vi "tensile_strength - Copy_debug.vi"(8 "Sampling rate":dbl=1000.0, 9 "error in (no error)":errorcluster, 10 "Sensor":tag="SimDev1/ai0:1", 11 "VISA Refnum in":refnum<visa-resource-name>) -> (1 "error out":errorcluster, 3 "VISA Refnum out":refnum<visa-resource-name>)   [LabVIEW 2020]
uses:
  <vilib>/DAQmx/read.llb/DAQmx Read (Analog 1D DBL NChan 1Samp).vi
  <vilib>/DAQmx/create/channels.llb/DAQmx Create Channel (AI-Voltage-Basic).vi
  <vilib>/DAQmx/configure/timing.llb/DAQmx Timing (Sample Clock).vi
  <vilib>/DAQmx/miscellaneous.llb/DAQmx Fill In Error Info.vi
panel:
  out "t = 3 - 0":dbl
  out "t = 1 - 0":dbl
  out "String":string
  in  "Lower limit for positioning":dbl
  out "distance value \n(changing)":dbl
  out "initial value(fixed)":dbl
  out "State indicator":u32
  in  "Upper limit for force":dbl
  in  "Upper limit for position":dbl
  in  "Emergency stop program(Long press)":bool
  out "Read":string
  in  "Stop motor":bool
  in  "Filename without ending":string="test"
  in  "File path":path=path "d:/temp"
  in  "Speed Write in mircometer/sec":string
  in  "Start Program":bool
  out "Numeric 3":i32
  in  "End the program":bool
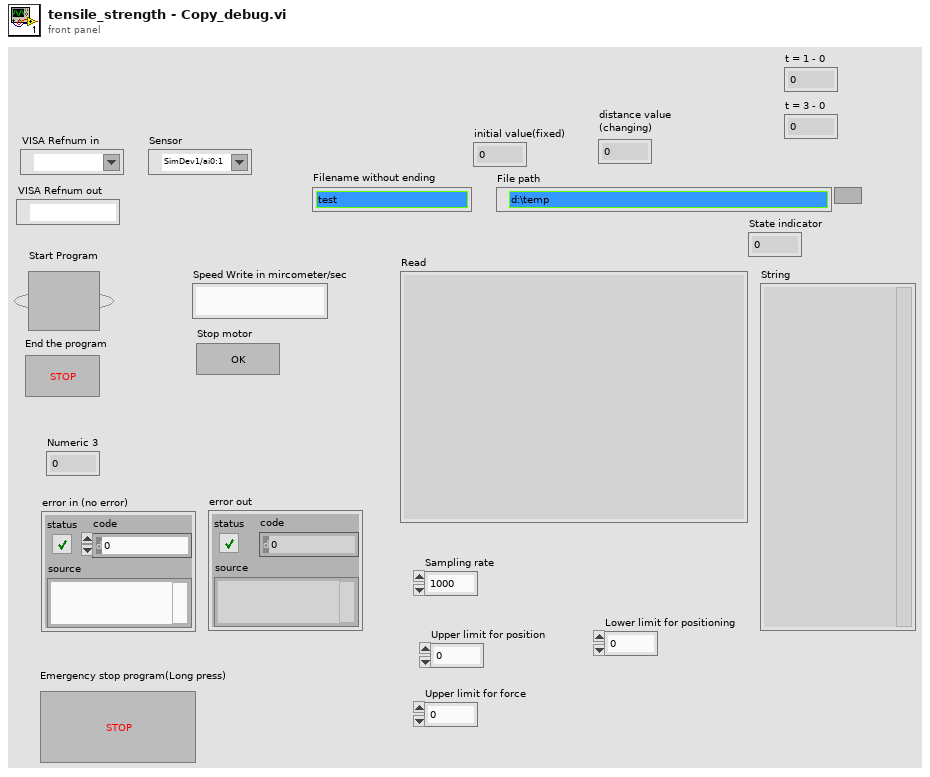
[diagram p1: front panel]
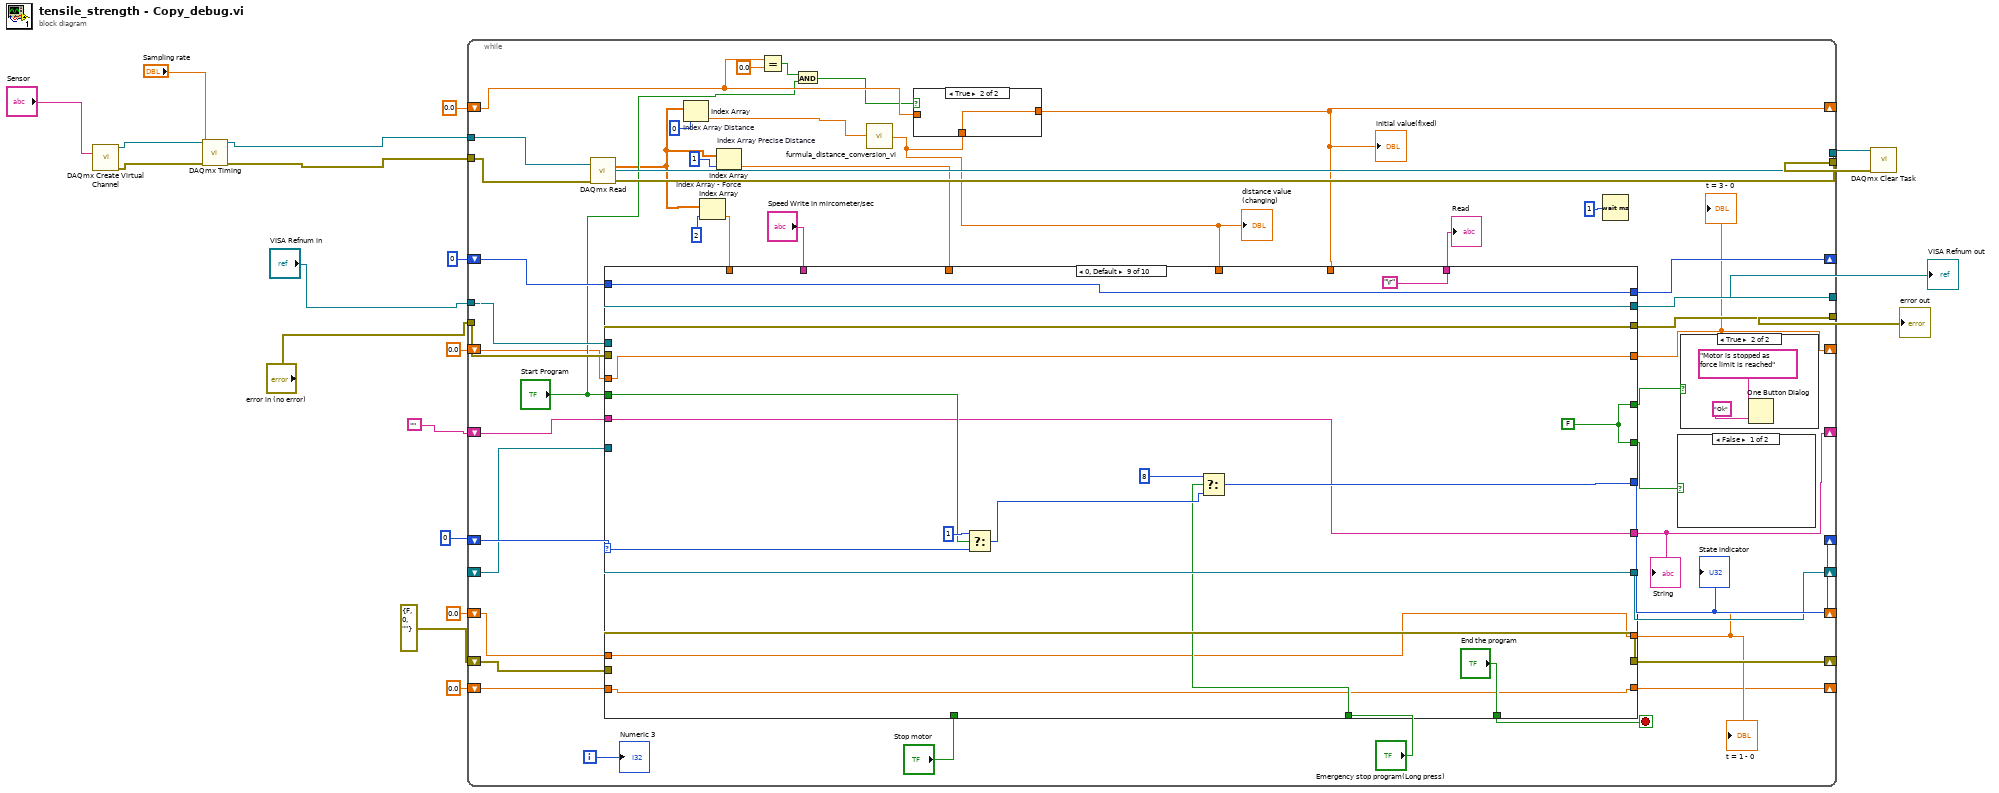
[diagram p0: block diagram]
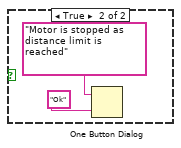
[diagram p2: hidden frame]
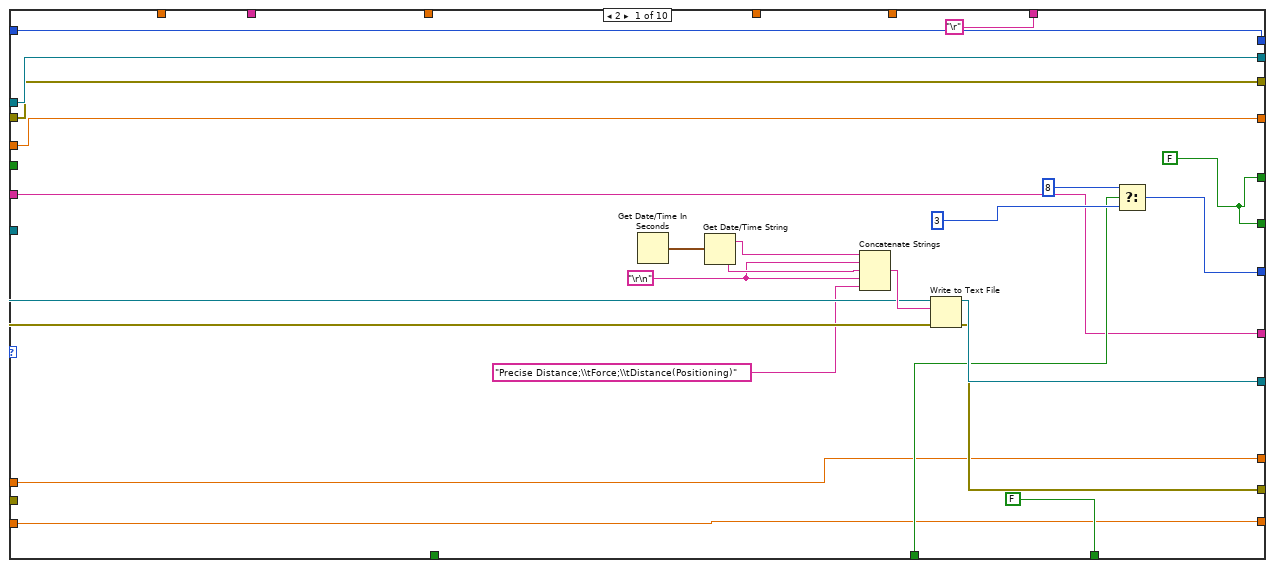
[diagram p5: hidden frame]
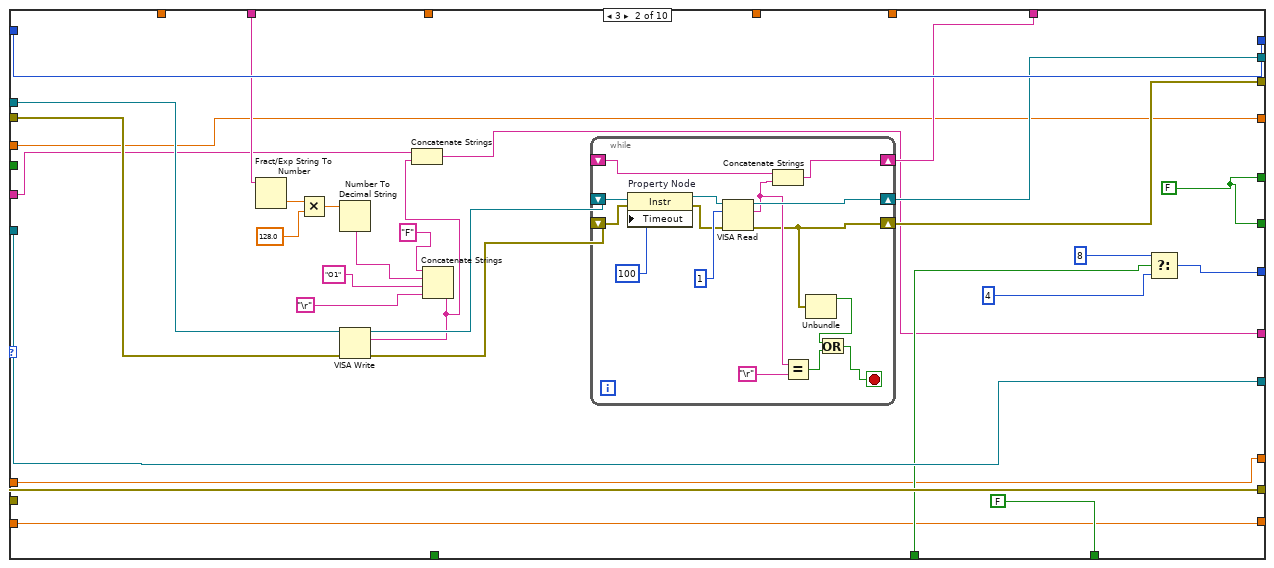
[diagram p6: hidden frame]
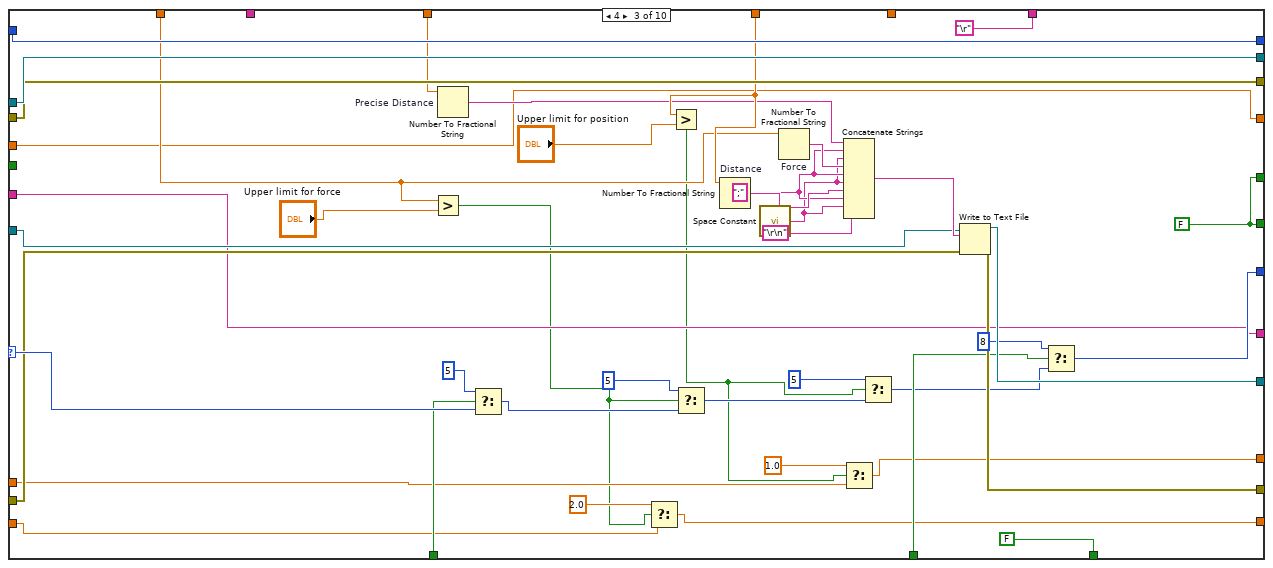
[diagram p7: hidden frame]
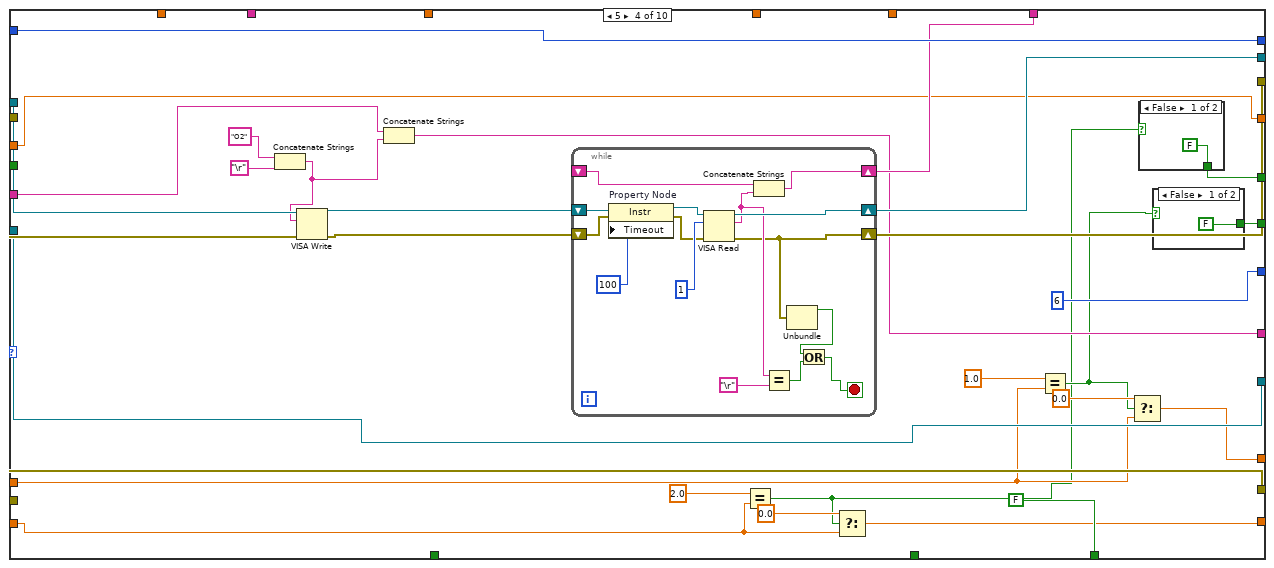
[diagram p8: hidden frame]
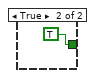
[diagram p9: hidden frame]
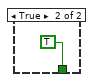
[diagram p10: hidden frame]
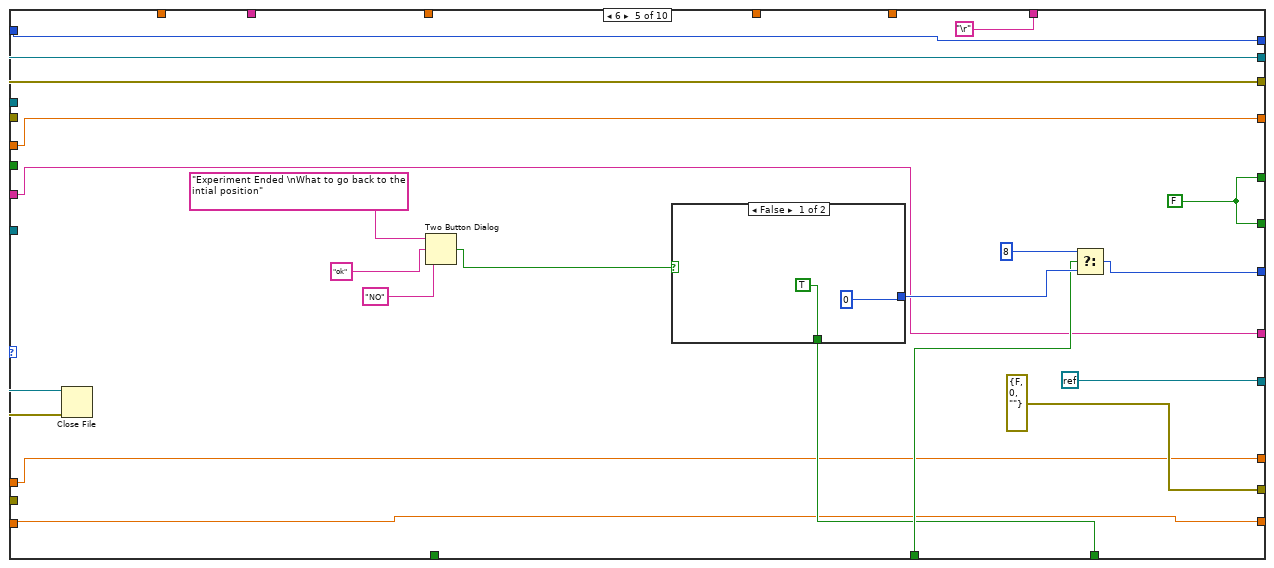
[diagram p11: hidden frame]
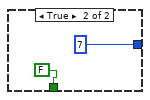
[diagram p12: hidden frame]
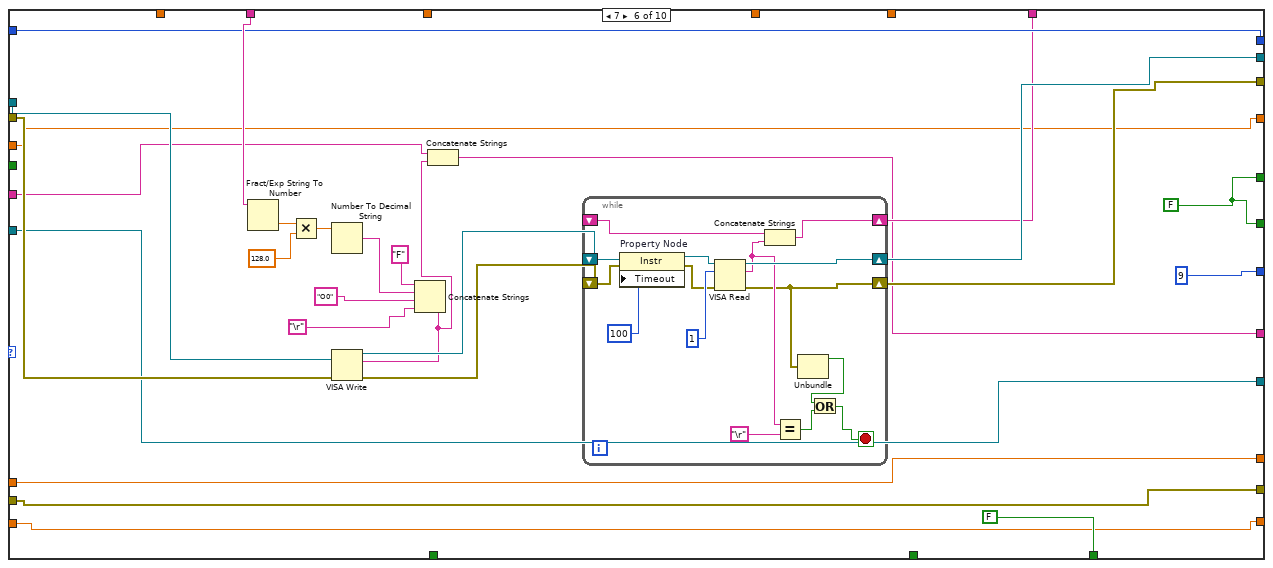
[diagram p13: hidden frame]
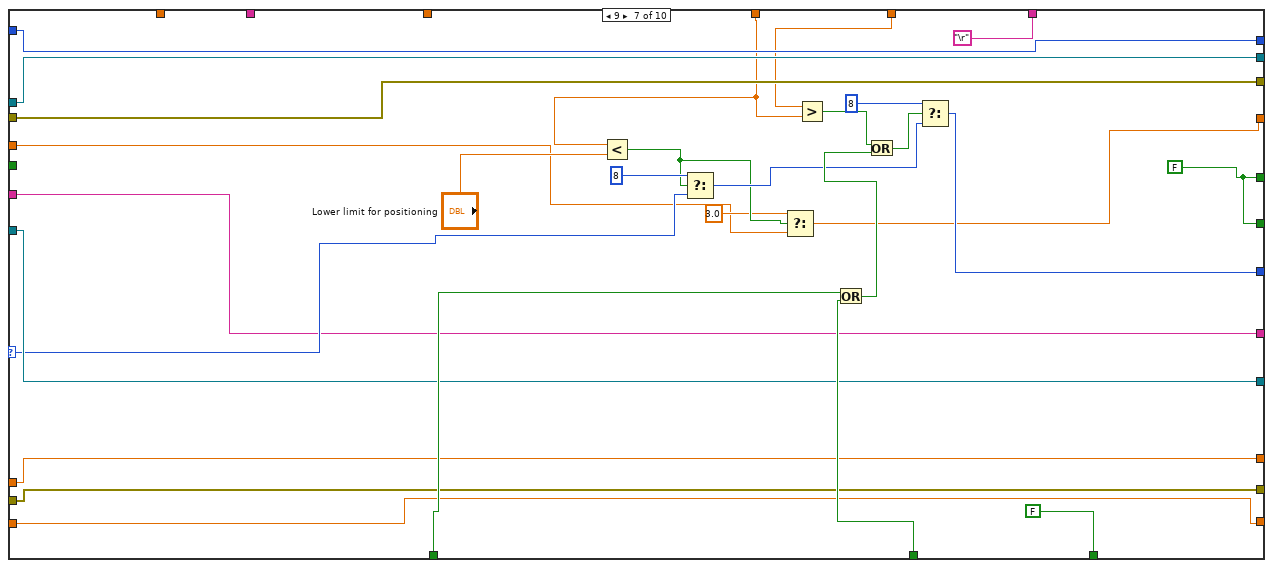
[diagram p14: hidden frame]
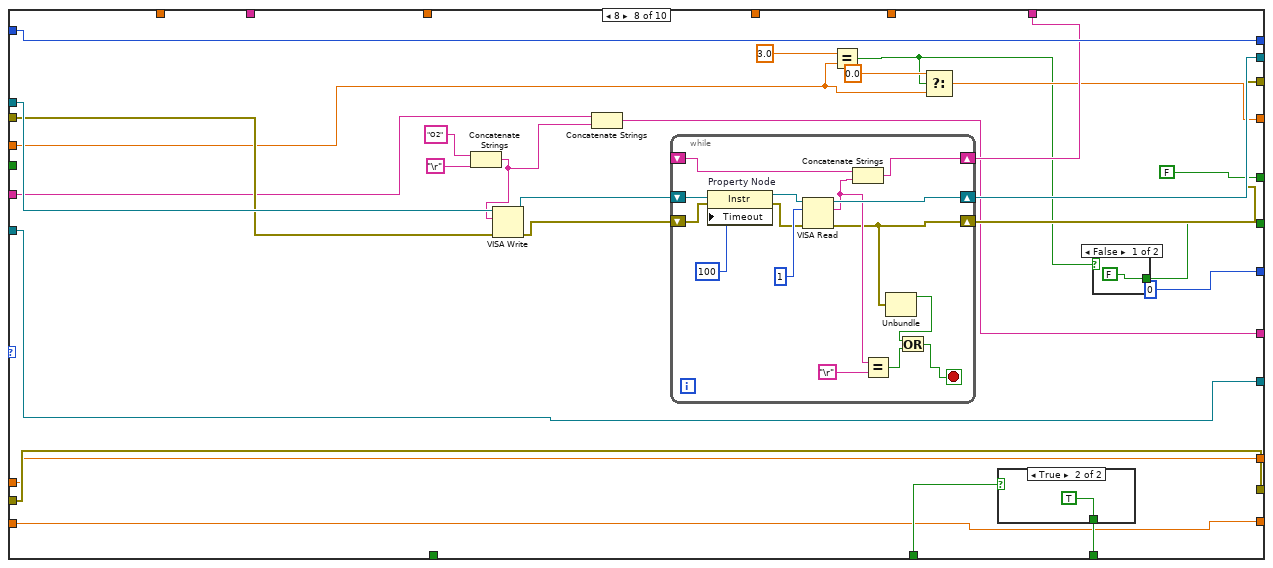
[diagram p15: hidden frame]
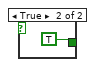
[diagram p16: hidden frame]
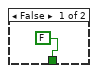
[diagram p17: hidden frame]
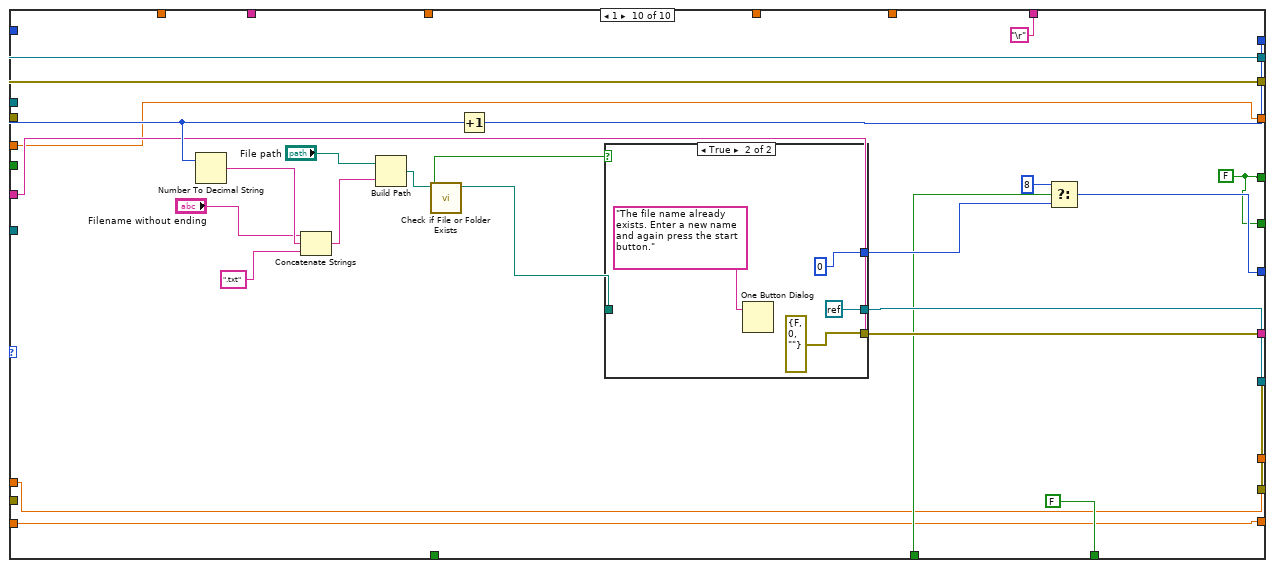
[diagram p18: hidden frame]
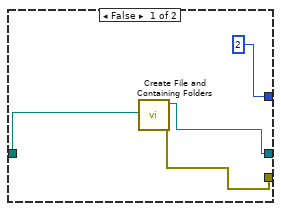
[diagram p19: hidden frame]
diagram:
  n1 = call-poly <vilib>:"DAQmx Create Virtual Channel.vi"("physical channels"="Sensor") -> ("task out"=w17:refnum<k21>, "error out"=w16:errorcluster)  [unwired: 13 in]
  n2 = call-poly <vilib>:"DAQmx Timing.vi"("task/channels in"=w17, "rate"="Sampling rate", "error in"=w16) -> ("task out"=w6:refnum<k21>, "error out"=w5:errorcluster)  [unwired: 11 in]
  n3 = while {
    tunnel: "VISA Refnum in" -> [w67]
    tunnel: "error in (no error)" -> [w66]
    tunnel: [w65] -> w8
    tunnel: [w64] -> w9
    shift-right: [w61] -> _
    shift-left: 0 -> [w63]
    shift-right: [w60] -> _
    shift-left: errorcluster {"status"=FALSE, "code"=0, "source"=""} ("error out") -> [w59]
    shift-right: [w58] -> _
    shift-left: 0 -> [w57]
    shift-right: [w56] -> _
    shift-left: _ -> [w55]
    tunnel: w6 -> [w53]
    tunnel: w5 -> [w54]
    tunnel: [w52] -> w15
    tunnel: [w51] -> w14
    shift-right: [w32] -> _
    shift-left: 0.0 -> [w46]
    shift-right: [w29] -> _
    shift-left: "" -> [w30]
    shift-right: [w28] -> _
    shift-left: 0.0 -> [w27]
    shift-right: [w26] -> _
    shift-left: 0.0 ("t") -> [w25]
    shift-right: [w24] -> _
    shift-left: 0.0 ("t") -> [w23]
    i -> [w62]
    stop <- w34 stop-if-true
    n4 = call-poly <vilib>:"DAQmx Read.vi"("task/channels in"=w53, "error in"=w54) -> ("task out"=w51:refnum<k21>, "data"=w37:dbl[], "error out"=w52:errorcluster)  [unwired: 11 in]
    n5 = Index Array "Index Array Distance"(array=w37, index=0) -> (element=w21:dbl)
    n6 = Index Array "Index Array - Force"(array=w37, index=2) -> (element=w47:dbl)
    n7 = Index Array "Index Array Precise Distance"(array=w37, index=1) -> (element=w35:dbl)
    n8 = Equal?(x=w46, y=0.0) -> (x = y?=w44:bool)
    n9 = And(x=w44, y="Start Program") -> (x .and. y?=w42:bool)
    n10 = call "furmula_distance_conversion_vi.vi"("Schieberegler"=w21) -> ("Numeric"=w22:dbl)
    "distance value \n(changing)" <- w22
    n11 = case shown="True" w42 {
      tunnel: w46 -> [w72 _]
      tunnel: w22 -> [_ w73]
      tunnel: [w72 w73] -> w32
      frame False {
      }
      frame True {
      }
    }
    "initial value(fixed)" <- w32
    n12 = case shown="0, Default" w63 {
      selector: w63 -> [_ _ w185 _ _ _ w313 _ w393 _]
      tunnel: w67 -> [w85 w127 w174 w214 w252 w282 w321 w353 w395 w408]
      tunnel: w66 -> [w84 w126 w173 w213 w251 w281 w320 w352 w394 w407]
      tunnel: [w84 w113 w173 w207 w251 w276 w320 w346 w394 w407] -> w65
      tunnel: [w85 w112 w174 w208 w252 w277 w321 w347 w395 w408] -> w64
      tunnel: [w81 w107 w154 u32 6 ("byte count") w242 9 w324 0 w384 w402] -> w61
      tunnel: [w89 w125 w178 w215 errorcluster {"status"=FALSE, "code"=0, "source"=""} ("error out") w278 w317 w349 w391 w409] -> w60
      tunnel: w59 -> [w91 w125 w177 w215 w256 w278 w317 w349 w391 _]
      tunnel: [FALSE FALSE FALSE FALSE w239 FALSE FALSE w344 "End the program" FALSE] -> w34
      tunnel: [w86 w122 w175 w206 w250 w275 w322 w351 w388 w412] -> w58
      tunnel: w57 -> [w86 w122 w175 w206 w250 w275 w322 w351 w388 w413]
      tunnel: [w90 w123 w179 w204 refnum<k0> refnum w279 w318 w350 w389 w410] -> w56
      tunnel: w55 -> [w92 w123 w172 w204 w255 w279 w318 w350 w389 _]
      tunnel: "Speed Write in mircometer/sec" -> [_ w118 _ _ _ w280 _ _ _ _]
      tunnel: w47 -> [_ _ w164 _ _ _ _ _ _ _]
      tunnel: w22 -> [_ _ w166 _ _ _ w303 _ _ _]
      tunnel: "Start Program" -> [_ _ _ _ _ _ _ _ w387 _]
      tunnel: w32 -> [_ _ _ _ _ _ w304 _ _ _]
      tunnel: ["\r" w111 "\r" w203 "\r" w273 "\r" w348 "\r" "\r"] -> w41
      tunnel: [w78 w106 w144 w197 w240 w267 w308 FALSE w381 w401] -> w40
      tunnel: "Stop motor" -> [_ _ w158 _ _ _ w326 _ _ _]
      tunnel: "Emergency stop program(Long press)" -> [w79 w109 w156 _ w241 _ w327 w343 w382 w404]
      tunnel: w35 -> [_ _ w165 _ _ _ _ _ _ _]
      tunnel: [w78 w106 w144 w193 w240 w267 w308 w332 w381 w401] -> w33
      tunnel: w30 -> [w77 w102 w153 w201 w238 w266 w312 w339 w380 w400]
      tunnel: [w77 w101 w153 w199 w238 w264 w312 w340 w380 w400] -> w29
      tunnel: [w76 w100 w152 w194 w237 w263 w311 w338 w379 w399] -> w28
      tunnel: w27 -> [w76 w100 w151 w195 w237 w263 w311 w338 w379 w399]
      tunnel: [w75 w99 w147 w189 w236 w262 w310 w337 w378 w398] -> w26
      tunnel: w25 -> [w75 w99 w146 w190 w236 w262 w310 w337 w378 w398]
      tunnel: [w74 w98 w143 w186 w235 w261 w306 w334 w377 w397] -> w24
      tunnel: w23 -> [w74 w98 w143 w186 w235 w261 w305 w331 w377 w397]
      frame 2 {
        w78 = FALSE
        w94 = "\r\n"
        n13 = Get Date/Time In Seconds() -> (seconds since 1Jan1904=w97:timestamp)
        n14 = Get Date/Time String(seconds (now)=w97) -> (date string=w96:string, time string=w95:string)  [unwired: 2 in]
        n15 = Concatenate Strings(w96, w94, w95, w94, "Precise Distance;\\tForce;\\tDistance(Positioning)" ("string")) -> (w93:string)
        n16 = Write to Text File(file (use dialog)=w92, text=w93, error in=w91) -> (refnum out=w90:refnum<file>, error out=w89:errorcluster)  [unwired: 1 in, 1 out]
        n17 = Select(t=8, s=w79, f=3) -> (s? t:f=w81:i32)
      }
      frame 3 {
        w106 = FALSE
        n18 = Fract/Exp String To Number(string=w118) -> (number=w120:dbl)  [unwired: 3 in, 1 out]
        n19 = Multiply(x=w120, y=128.0) -> (x*y=w121:dbl)
        n20 = Number To Decimal String(number=w121) -> (decimal integer string=w105:string)  [unwired: 1 in]
        n21 = Concatenate Strings("F" ("string"), w105, "O1" ("string"), "\r") -> (w103:string)
        n22 = VISA Write(VISA resource name=w127, write buffer=w103, error in (no error)=w126) -> (VISA resource name out=w114:refnum<visa-resource-name>, error out=w115:errorcluster)  [unwired: 1 out]
        n23 = Concatenate Strings(w102, w103) -> (w101:string)
        n24 = while {
          shift-right: [w129] -> w113
          shift-left: w115 -> [w132]
          shift-right: [w142] -> w112
          shift-left: w114 -> [w134]
          shift-right: [w139] -> w111
          shift-left: _ -> [w140]
          stop <- w135 stop-if-true
          n25 = property on="Property Node" class="Instr"(reference=w134, error in=w132, "Timeout"=u32 100 ("General Settings:Timeout Value")) -> (reference out=w133:refnum<visa-resource-name>, error out=w131:errorcluster)
          n26 = VISA Read(VISA resource name=w133, byte count=u32 1, error in (no error)=w131) -> (VISA resource name out=w142:refnum<visa-resource-name>, read buffer=w138:string, error out=w129:errorcluster)  [unwired: 1 out]
          n27 = Concatenate Strings(w140, w138) -> (w139:string)
          n28 = Equal?(x=w138, y="\r") -> (x = y?=w136:bool)
          n29 = Unbundle(w129) -> ("status"=w128:bool)  [unwired: 2 out]
          n30 = Or(x=w128, y=w136) -> (x .or. y?=w135:bool)
        }
        n31 = Select(t=8, s=w109, f=u32 4 ("byte count")) -> (s? t:f=w107:u32)
      }
      frame 4 {
        w144 = FALSE
        w162 = ";"
        n32 = Greater?(x=w164, y="Upper limit for force") -> (0:w145:bool)
        n33 = Number To Fractional String "Precise Distance"(number=w165) -> (F-format string=w163:string)  [unwired: 3 in]
        n34 = Select(t=u32 5, s=w158, f=w185) -> (s? t:f=w171:u32)
        n35 = Select(t=2.0, s=w145, f=w146) -> (s? t:f=w147:dbl)
        n36 = Greater?(x=w166, y="Upper limit for position") -> (0:w149:bool)
        n37 = Select(t=u32 5, s=w145, f=w171) -> (s? t:f=w170:u32)
        n38 = Number To Fractional String "Distance"(number=w166) -> (F-format string=w182:string)  [unwired: 3 in]
        n39 = call <vilib>:"Space Constant.vi"() -> ("String"=w161:string)
        n40 = Number To Fractional String "Force"(number=w164) -> (F-format string=w183:string)  [unwired: 3 in]
        n41 = Concatenate Strings(w163, w162, w161, w183, w162, w161, w182, w162, w161, "\r\n") -> (w180:string)
        n42 = Select(t=1.0, s=w149, f=w151) -> (s? t:f=w152:dbl)
        n43 = Select(t=u32 5, s=w149, f=w170) -> (s? t:f=w155:u32)
        n44 = Write to Text File(file (use dialog)=w172, text=w180, error in=w177) -> (refnum out=w179:refnum<file>, error out=w178:errorcluster)  [unwired: 1 in, 1 out]
        n45 = Select(t=8, s=w156, f=w155) -> (s? t:f=w154:u32)
      }
      frame 5 {
        n46 = Concatenate Strings("O2" ("write buffer"), "\r") -> (w200:string)
        n47 = VISA Write(VISA resource name=w214, write buffer=w200, error in (no error)=w213) -> (VISA resource name out=w211:refnum<visa-resource-name>, error out=w212:errorcluster)  [unwired: 1 out]
        n48 = Concatenate Strings(w201, w200) -> (w199:string)
        n49 = while {
          shift-right: [w221] -> w207
          shift-left: w212 -> [w224]
          shift-right: [w234] -> w208
          shift-left: w211 -> [w226]
          shift-right: [w231] -> w203
          shift-left: _ -> [w232]
          stop <- w227 stop-if-true
          n50 = property on="Property Node" class="Instr"(reference=w226, error in=w224, "Timeout"=u32 100 ("General Settings:Timeout Value")) -> (reference out=w225:refnum<visa-resource-name>, error out=w223:errorcluster)
          n51 = VISA Read(VISA resource name=w225, byte count=u32 1, error in (no error)=w223) -> (VISA resource name out=w234:refnum<visa-resource-name>, read buffer=w230:string, error out=w221:errorcluster)  [unwired: 1 out]
          n52 = Concatenate Strings(w232, w230) -> (w231:string)
          n53 = Equal?(x=w230, y="\r") -> (x = y?=w228:bool)
          n54 = Unbundle(w221) -> ("status"=w220:bool)  [unwired: 2 out]
          n55 = Or(x=w220, y=w228) -> (x .or. y?=w227:bool)
        }
        n56 = Equal?(x=2.0, y=w190) -> (x = y?=w187:bool)
        n57 = Select(t=0.0, s=w187, f=w190) -> (s? t:f=w189:dbl)
        n58 = Equal?(x=1.0, y=w195) -> (x = y?=w188:bool)
        n59 = Select(t=0.0, s=w188, f=w195) -> (s? t:f=w194:dbl)
        n60 = case shown="False" w187 {
          tunnel: [FALSE TRUE] -> w197
          frame False {
          }
          frame True {
          }
        }
        n61 = case shown="False" w188 {
          tunnel: [FALSE TRUE] -> w193
          frame False {
          }
          frame True {
          }
        }
      }
      frame 6 {
        w240 = FALSE
        n62 = Close File(refnum=w255, error in=w256) -> ()  [unwired: 2 out]
        n63 = Two Button Dialog(message="Experiment Ended \nWhat to go back to the intial position", 1:"NO" ("F button name (\"Cancel\")"), 2:"ok" ("T button name (\"OK\")")) -> (T button?=w245:bool)
        n64 = case shown="False" w245 {
          tunnel: [u32 0 ("byte count") u32 7 ("byte count")] -> w243
          tunnel: [TRUE FALSE] -> w239
          frame False {
          }
          frame True {
          }
        }
        n65 = Select(t=8, s=w241, f=w243) -> (s? t:f=w242:u32)
      }
      frame 7 {
        w267 = FALSE
        n66 = Fract/Exp String To Number(string=w280) -> (number=w286:dbl)  [unwired: 3 in, 1 out]
        n67 = Multiply(x=w286, y=128.0) -> (x*y=w287:dbl)
        n68 = Number To Decimal String(number=w287) -> (decimal integer string=w268:string)  [unwired: 1 in]
        n69 = Concatenate Strings("F" ("string"), w268, "O0" ("string"), "\r") -> (w265:string)
        n70 = VISA Write(VISA resource name=w282, write buffer=w265, error in (no error)=w281) -> (VISA resource name out=w283:refnum<visa-resource-name>, error out=w284:errorcluster)  [unwired: 1 out]
        n71 = Concatenate Strings(w266, w265) -> (w264:string)
        n72 = while {
          shift-right: [w289] -> w276
          shift-left: w284 -> [w292]
          shift-right: [w302] -> w277
          shift-left: w283 -> [w294]
          shift-right: [w299] -> w273
          shift-left: _ -> [w300]
          stop <- w295 stop-if-true
          n73 = property on="Property Node" class="Instr"(reference=w294, error in=w292, "Timeout"=u32 100 ("General Settings:Timeout Value")) -> (reference out=w293:refnum<visa-resource-name>, error out=w291:errorcluster)
          n74 = VISA Read(VISA resource name=w293, byte count=u32 1, error in (no error)=w291) -> (VISA resource name out=w302:refnum<visa-resource-name>, read buffer=w298:string, error out=w289:errorcluster)  [unwired: 1 out]
          n75 = Concatenate Strings(w300, w298) -> (w299:string)
          n76 = Equal?(x=w298, y="\r") -> (x = y?=w296:bool)
          n77 = Unbundle(w289) -> ("status"=w288:bool)  [unwired: 2 out]
          n78 = Or(x=w288, y=w296) -> (x .or. y?=w295:bool)
        }
      }
      frame 9 {
        w308 = FALSE
        n79 = Less?(x=w303, y="Lower limit for positioning") -> (x < y?=w309:bool)
        n80 = Select(t=u32 8, s=w309, f=w313) -> (s? t:f=w315:u32)
        n81 = Select(t=3.0, s=w309, f=w305) -> (s? t:f=w306:dbl)
        n82 = Greater?(x=w304, y=w303) -> (0:w329:bool)
        n83 = Or(x=w326, y=w327) -> (x .or. y?=w325:bool)
        n84 = Or(x=w329, y=w325) -> (x .or. y?=w328:bool)
        n85 = Select(t=u32 8, s=w328, f=w315) -> (s? t:f=w324:u32)
      }
      frame 8 {
        n86 = Concatenate Strings("O2" ("write buffer"), "\r") -> (w341:string)
        n87 = VISA Write(VISA resource name=w353, write buffer=w341, error in (no error)=w352) -> (VISA resource name out=w356:refnum<visa-resource-name>, error out=w357:errorcluster)  [unwired: 1 out]
        n88 = Concatenate Strings(w339, w341) -> (w340:string)
        n89 = while {
          shift-right: [w363] -> w346
          shift-left: w357 -> [w366]
          shift-right: [w376] -> w347
          shift-left: w356 -> [w368]
          shift-right: [w373] -> w348
          shift-left: _ -> [w374]
          stop <- w369 stop-if-true
          n90 = property on="Property Node" class="Instr"(reference=w368, error in=w366, "Timeout"=u32 100 ("General Settings:Timeout Value")) -> (reference out=w367:refnum<visa-resource-name>, error out=w365:errorcluster)
          n91 = VISA Read(VISA resource name=w367, byte count=u32 1, error in (no error)=w365) -> (VISA resource name out=w376:refnum<visa-resource-name>, read buffer=w372:string, error out=w363:errorcluster)  [unwired: 1 out]
          n92 = Concatenate Strings(w374, w372) -> (w373:string)
          n93 = Equal?(x=w372, y="\r") -> (x = y?=w370:bool)
          n94 = Unbundle(w363) -> ("status"=w362:bool)  [unwired: 2 out]
          n95 = Or(x=w362, y=w370) -> (x .or. y?=w369:bool)
        }
        n96 = Equal?(x=3.0, y=w331) -> (x = y?=w333:bool)
        n97 = Select(t=0.0, s=w333, f=w331) -> (s? t:f=w334:dbl)
        n98 = case shown="True" w343 {
          tunnel: [FALSE TRUE] -> w344
          frame False {
          }
          frame True {
          }
        }
        n99 = case shown="False" w333 {
          tunnel: [FALSE TRUE] -> w332
          frame False {
          }
          frame True {
          }
        }
      }
      frame 0, Default {
        w381 = FALSE
        n100 = Select(t=1, s=w387, f=w393) -> (s? t:f=w385:u32)
        n101 = Select(t=u32 8, s=w382, f=w385) -> (s? t:f=w384:u32)
      }
      frame 1 {
        w401 = FALSE
        n102 = Number To Decimal String(number=w413) -> (decimal integer string=w417:string)  [unwired: 1 in]
        n103 = Concatenate Strings("Filename without ending", w417, ".txt") -> (w416:string)
        n104 = Build Path(base path="File path", name or relative path=w416) -> (appended path=w418:path)
        n105 = call <vilib>:"Check if File or Folder Exists.vi"("path"=w418) -> ("file or folder exists?"=w419:bool, "dup path"=w420:path)  [unwired: 8 in, 1 out]
        n106 = Increment(x=w413) -> (x+1=w412:i32)
        n107 = case shown="True" w419 {
          tunnel: w420 -> [w423 _]
          tunnel: [w421 errorcluster {"status"=FALSE, "code"=0, "source"=""} ("Fehlerkonstante")] -> w409
          tunnel: [w422 refnum<k0> refnum] -> w410
          tunnel: [2 ("f") 0] -> w405
          frame False {
            n108 = call <vilib>:"Create File and Containing Folders.vi"("file path"=w423) -> ("error out"=w421:errorcluster, "refnum out"=w422:refnum<file>)  [unwired: 9 in]
          }
          frame True {
            n109 = One Button Dialog(message="The file name already exists. Enter a new name and again press the start button.") -> ()  [unwired: 1 in, 1 out]
          }
        }
        n110 = Select(t=8, s=w404, f=w405) -> (s? t:f=w402:i32)
      }
    }
    "Read" <- w41
    "State indicator" <- w61
    "String" <- w29
    "t = 1 - 0" <- w28
    "t = 3 - 0" <- w24
    n111 = Wait (ms)(milliseconds to wait=u32 1 ("Zu wartende ms")) -> ()  [unwired: 1 out]
    n112 = case shown="False" w33 {
      frame False {
      }
      frame True {
        n113 = One Button Dialog(message="Motor is stopped as  distance limit is reached", button name ("OK")="Ok") -> ()  [unwired: 1 out]
      }
    }
    n114 = case shown="True" w40 {
      frame False {
      }
      frame True {
        n115 = One Button Dialog(message="Motor is stopped as  force limit is reached", button name ("OK")="Ok") -> ()  [unwired: 1 out]
      }
    }
    "Numeric 3" <- w62
  }
  "VISA Refnum out" <- w9
  "error out" <- w8
  n116 = call <vilib>:"DAQmx Clear Task.vi"("task in"=w14, "error in"=w15) -> ()  [unwired: 13 in, 1 out]
